vi "Example Simple.vi"() -> ()   [LabVIEW 2010]
uses:
  C:/tf/play/labview/Tinkerforge.dll
  Tinkerforge.dll
panel:
  out "pm10.0 (µg/m³)":i32
  out "pm2.5 (µg/m³)":i32
  out "pm1.0 (µg/m³)":i32
  in  "uid":string="abc"
  in  "port":i32=4223
  in  "host":string="localhost"
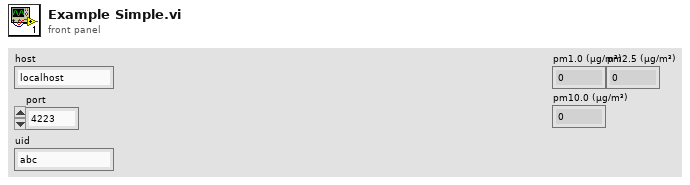
[diagram p1: front panel]
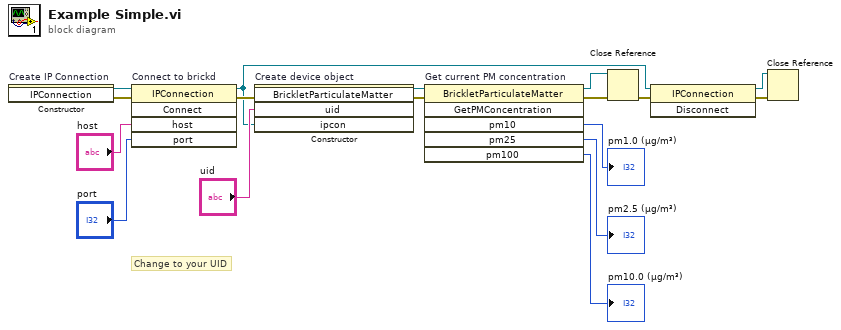
[diagram p0: block diagram]
diagram:
  # "Change to your UID"
  n1 = constructor on="Create IP Connection" class="IPConnection"() -> (reference out=w17:refnum<k24>, error out=w4:errorcluster)  [unwired: 3 in, 1 out]
  n2 = invoke on="Connect to brickd" class="IPConnection" method="Connect"(reference=w17, error in=w4, "host"="host", "port"="port") -> (reference out=w6:refnum<k24>, error out=w13:errorcluster)  [unwired: 1 in, 3 out]
  n3 = constructor on="Create device object" class="BrickletParticulateMatter"(error in=w13, "uid"="uid", "ipcon"=w6) -> (reference out=w11:refnum<k24>, error out=w12:errorcluster)  [unwired: 2 in, 3 out]
  n4 = invoke on="Get current PM concentration" class="BrickletParticulateMatter" method="GetPMConcentration"(reference=w11, error in=w12) -> (reference out=w9:refnum<k24>, error out=w10:errorcluster, "pm10"=→"pm1.0 (µg/m³)":i32, "pm25"=→"pm2.5 (µg/m³)":i32, "pm100"=→"pm10.0 (µg/m³)":i32)  [unwired: 4 in, 1 out]
  n5 = Close Reference(reference=w9, error in (no error)=w10) -> (error out=w8:errorcluster)
  n6 = invoke class="IPConnection" method="Disconnect"(reference=w6, error in=w8) -> (reference out=w5:refnum<k24>, error out=w7:errorcluster)  [unwired: 1 in, 1 out]
  n7 = Close Reference(reference=w5, error in (no error)=w7) -> ()  [unwired: 1 out]
